vi "Read Meta Data.vi"(7 "Linked List ID":string, 8 "error in (no error)":errorcluster, 11 "Linked List in":refnum<class "Linked List.lvclass">) -> (0 "error out":errorcluster, 1 "Found?":bool, 2 "Meta Data":string, 3 "Linked List out":refnum<class "Linked List.lvclass">)   [LabVIEW 2019, in "Linked Lists.lvlib" / "Linked List.lvclass"]
uses:
  <vilib>/gpm_packages/@cs/linked-list/Source/Linked List/Linked List/Linked List.lvclass
  <vilib>/gpm_packages/@cs/linked-list/Source/Linked List/Linked List Definition/Linked List Definition.lvclass
  <vilib>/gpm_packages/@cs/linked-list/Source/Linked List/Linked List/Linked List.lvclass/Linked List.ctl
  <vilib>/gpm_packages/@cs/lookup-table/Source/LookupTable/LookupTable.lvclass/LookupTable.ctl
  44476107-6b6d-492f-8275-d8162641636c.vi
  <vilib>/gpm_packages/@cs/lookup-table/Source/LookupTable/Read Table Reference.vi
  44476107-6b6d-492f-8275-d8162641636c.vi/1ee4e8ad-1344-49e5-bbff-1ee0841a379b.vi
  <vilib>/gpm_packages/@cs/lookup-table/Source/LookupTable/LookupTable.lvclass
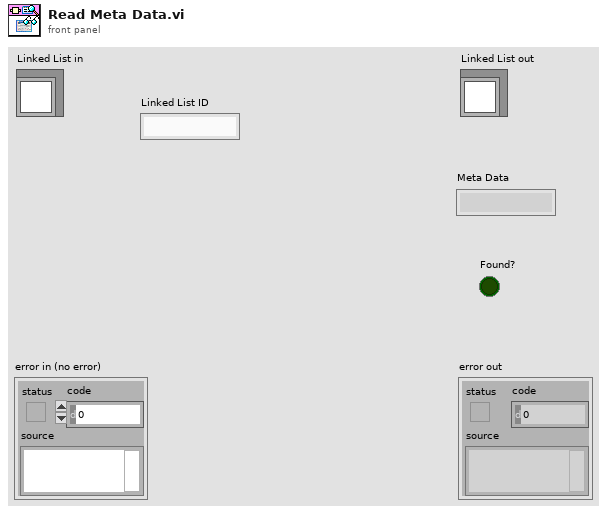
[diagram p1: front panel]
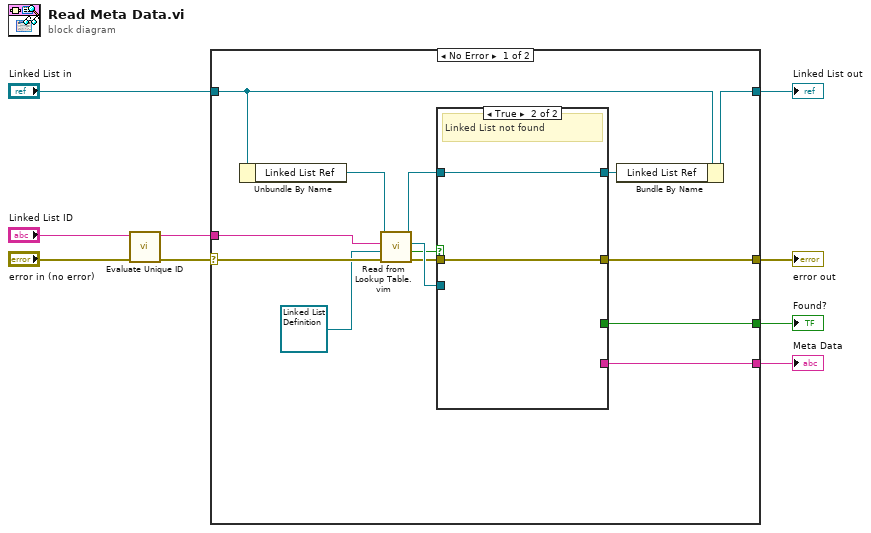
[diagram p0: block diagram]
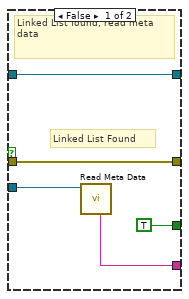
[diagram p2: hidden frame]
diagram:
  n1 = call <vilib>:"Evaluate Unique ID.vi"("error in (no error)"="error in (no error)", "Unique ID"="Linked List ID") -> ("error out"=w7:errorcluster, "Unique ID Out"=w6:string)  [unwired: 8 in]
  n2 = case shown="No Error" w7 {
    selector: w7 -> [w22 w31]
    tunnel: w6 -> [w23 _]
    tunnel: [w17 w32] -> w5
    tunnel: "Linked List in" -> [w18 w32]
    tunnel: [w11 w31] -> w3
    tunnel: [w16 _] -> w2
    tunnel: [w10 _] -> w1
    frame No Error {
      n3 = Unbundle By Name(w18) -> ("Linked List Ref"=w20:refnum<data-value>)
      n4 = call "Read from Lookup Table.vim"("error in (no error)"=w22, "Type"=refnum<class "Linked List Definition.lvclass"> refnum ("Linked List.lvlib:Linked List Definition.lvclass"), "Item Name"=w23, "LookupTable Reference"=w20) -> ("error out"=w12:errorcluster, "Not Found?"=w13:bool, "Value"=w19:refnum<class "Linked List Definition.lvclass">, "LookupTable Reference Out"=w15:refnum<data-value>)  [unwired: 4 in]
      n5 = case shown="True" w13 {
        tunnel: w19 -> [w28 _]
        tunnel: [w27 _] -> w16
        tunnel: [w26 w30] -> w14
        tunnel: w15 -> [w26 w30]
        tunnel: w12 -> [w25 w29]
        tunnel: [w25 w29] -> w11
        tunnel: [TRUE _] -> w10
        frame False {
          # "Linked List Found"
          # "Linked List found, read meta data"
          n6 = call <vilib>:"Read Meta Data.vi"("Linked List Definition in"=w28) -> ("Meta Data"=w27:string)  [unwired: 9 in, 1 out]
        }
        frame True {
          # "Linked List not found"
        }
      }
      n7 = Bundle By Name(cluster=w18, "Linked List Ref"=w14) -> (w17:refnum<class "Linked List.lvclass">)
    }
    frame Error {
    }
  }
  "error out" <- w3
  "Linked List out" <- w5
  "Found?" <- w1
  "Meta Data" <- w2
